vi "Instrument Manager Loop.vi"(8 "System Control":refnum<queue>, 11 "Instrument Manager":refnum<queue>) -> (0 "error out":errorcluster)   [LabVIEW 2020, in "Omega Platinum Series Plugin.lvlib" / "Instrument Manager.lvlib"]
uses:
  Instrument Manager/Instrument Manager.lvlib
  support/Message Queue/Message Cluster.ctl
  Instrument Manager/Instrument State.ctl
  <vilib>/Utility/error.llb/Error Cluster From Error Code.vi
  <vilib>/ErrorRing/Error Ring.xnode
  support/Message Queue/Message Queue.lvlib
  Omega Platinum Series Plugin.lvlib
  <instrlib>/RxnRover/OmegaPlatinumSeriesDriver/Omega Platinum Series.lvlib
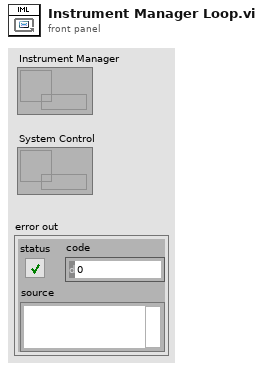
[diagram p1: front panel]
types:
  T1 = typedef "Omega Platinum Series Plugin.lvlib/Instrument Manager.lvlib/Instrument State.ctl" = cluster{"VISA Resource":refnum<visa-resource-name>, "Setpoint":dbl, "Running":bool, "Running Since":timestamp, "Data Point":cluster{"Time Stamp":timestamp, "Value":dbl}, "Sampling Rate (sec/sample)":dbl}
  T2 = typedef "Omega Platinum Series.lvlib/System State.ctl" = enum16{"LOAD", "IDLE", "INPUT_ADJUST", "CONTROL_ADJUST", "MODIFY", "WAIT", "RUN", "STANDBY", "STOP", "PAUSE", "FAULT", "SHUTDOWN", "AUTOTUNE"}
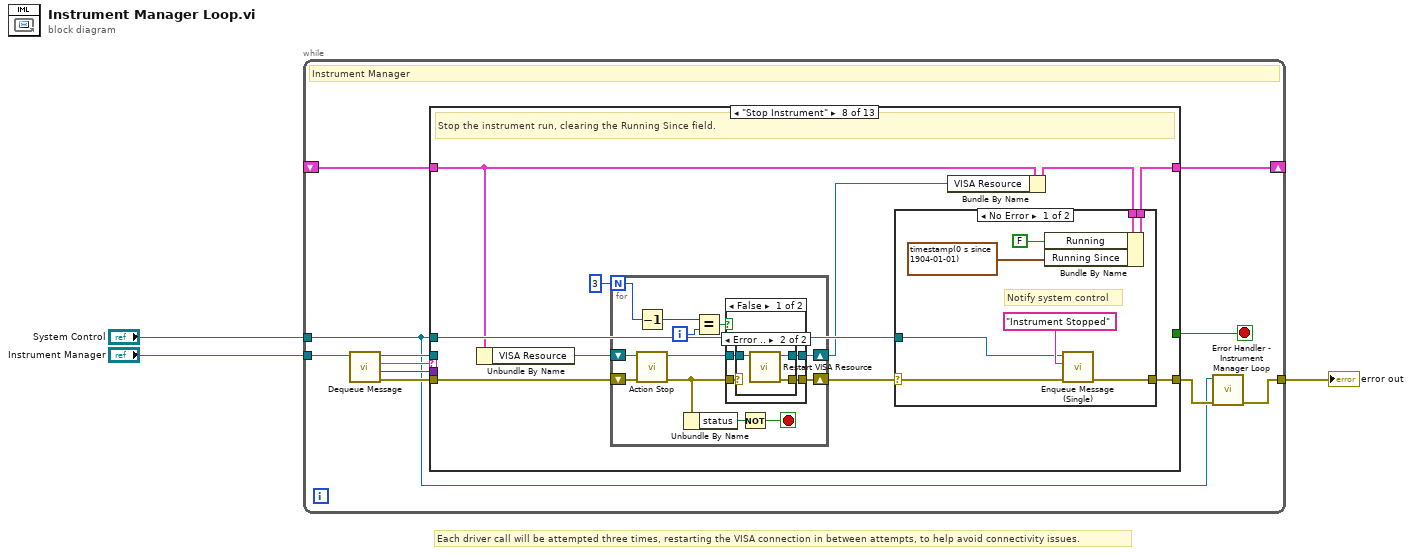
[diagram p0: block diagram]
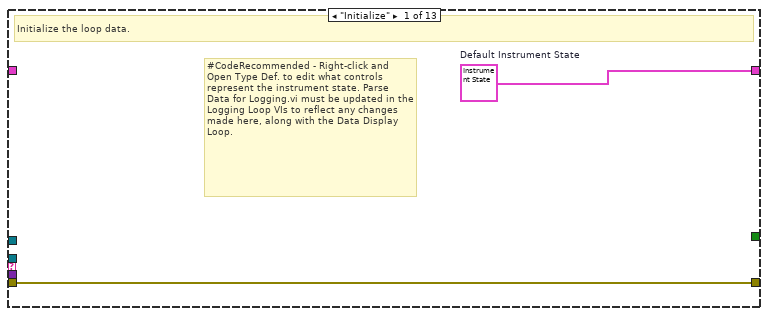
[diagram p2: hidden frame]
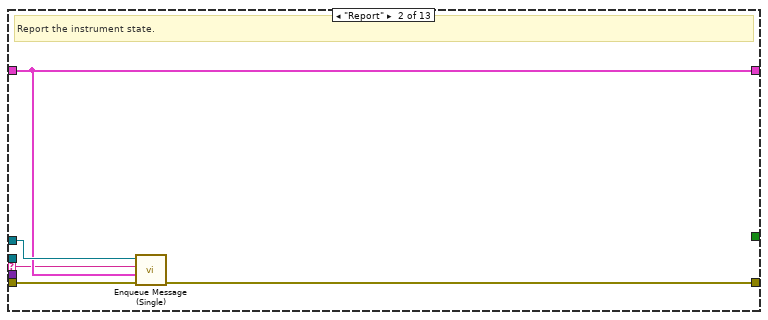
[diagram p3: hidden frame]
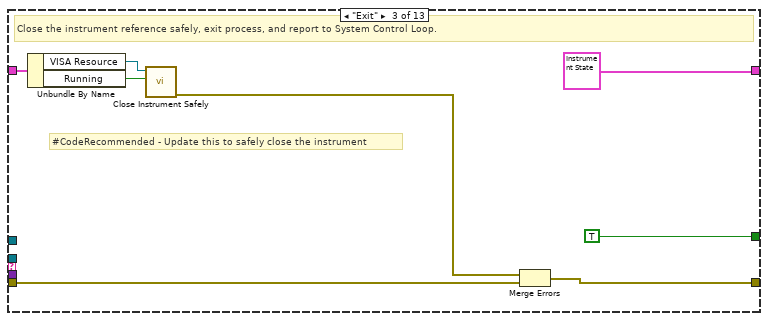
[diagram p4: hidden frame]
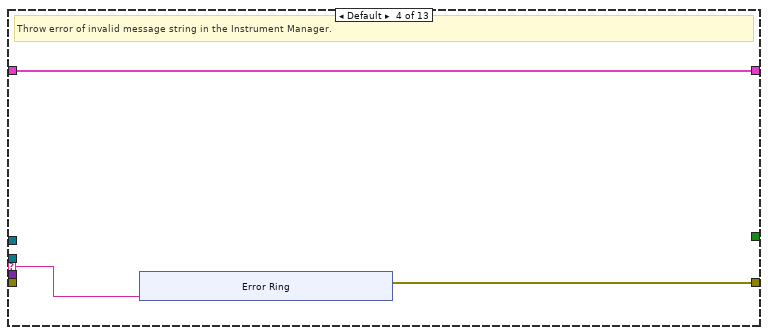
[diagram p5: hidden frame]
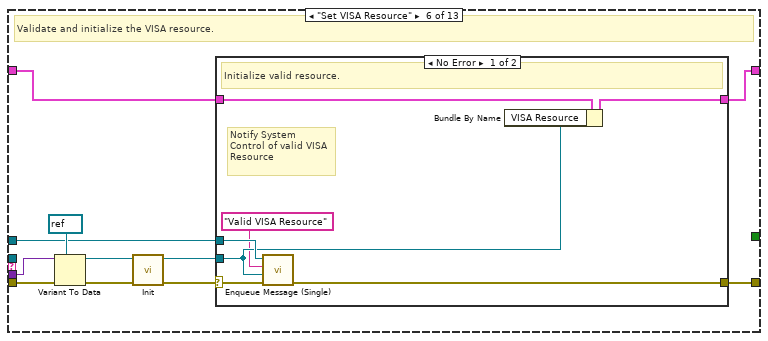
[diagram p7: hidden frame]
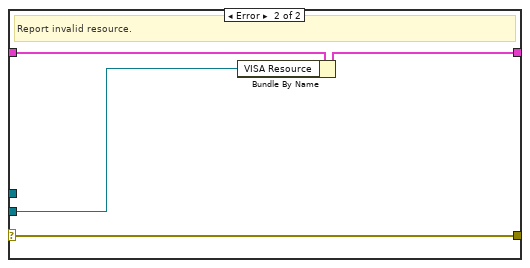
[diagram p8: hidden frame]
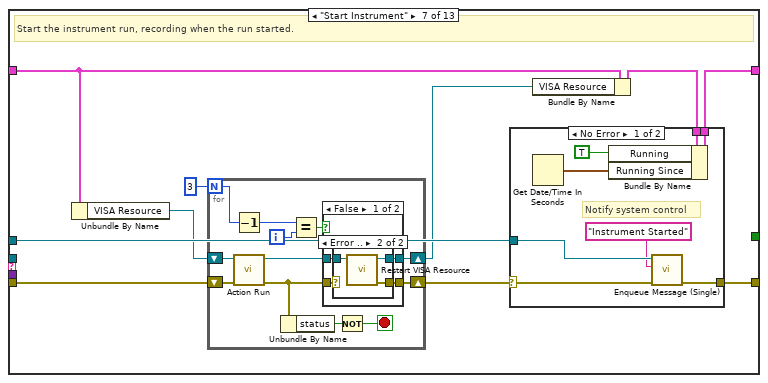
[diagram p9: hidden frame]
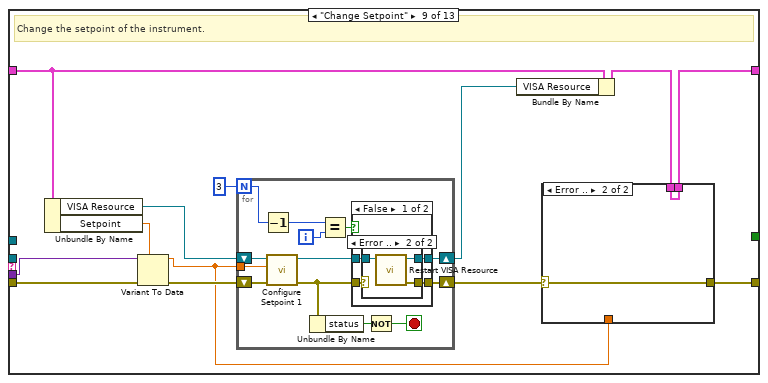
[diagram p16: hidden frame]
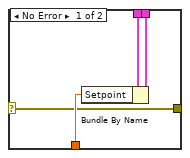
[diagram p17: hidden frame]
diagram:
  # "Each driver call will be attempted three times, restarting the VISA connection in between attempts, to help avoid connectivity issues."
  n1 = while {
    tunnel: "Instrument Manager" -> [w14]
    tunnel: "System Control" -> [w5]
    tunnel: [w8] -> w1
    shift-right: [w7] -> _
    shift-left: _ -> [w4]
    stop <- w6 stop-if-true
    # "Instrument Manager"
    n2 = call "Dequeue Message.vi"("Message Queue"=w14) -> ("error out"=w10:errorcluster, "Message Data"=w11:variant, "Message"=w13:string, "dup Message Queue"=w12:refnum<queue>)  [unwired: 7 in]
    n3 = case shown="\"Stop Instrument\"" w13 {
      selector: w13 -> [_ w17 _ w31 _ _ _ _ _ _ _ _ _]
      tunnel: w12 -> [_ _ _ _ _ _ _ _ _ _ _ _ _]
      tunnel: w5 -> [_ w20 _ _ _ w42 w72 w115 _ _ _ _ _]
      tunnel: w11 -> [_ _ _ _ _ w49 _ _ w161 _ _ _ _]
      tunnel: w10 -> [w15 w21 w24 _ w40 w48 w68 w112 w156 w194 w203 w239 w284]
      tunnel: [w15 w19 w23 w30 w40 w52 w73 w116 w152 w194 w202 w237 w280] -> w9
      tunnel: w4 -> [_ w18 w29 w32 w41 w51 w70 w113 w160 w193 w197 w236 w279]
      tunnel: [w16 w18 T1 {"VISA Resource"="", "Setpoint"=0.0, "Running"=FALSE, "Running Since"=timestamp(0 s since 1904-01-01), "Data Point"={"Time Stamp"=timestamp(0 s since 1904-01-01), "Value"=0.0}, "Sampling Rate (sec/sample)"=0.0} w32 w41 w50 w71 w114 w162 w193 w199 w243 w286] -> w7
      tunnel: [_ _ TRUE _ _ _ _ _ _ _ _ _ _] -> w6
      frame "Initialize" {
        w16 = T1 {"VISA Resource"="", "Setpoint"=0.0, "Running"=FALSE, "Running Since"=timestamp(0 s since 1904-01-01), "Data Point"={"Time Stamp"=timestamp(0 s since 1904-01-01), "Value"=0.0}, "Sampling Rate (sec/sample)"=0.0}  # Default Instrument State
        # "#CodeRecommended - Right-click and Open Type Def. to edit what controls represent the instrument state. Parse Data for Logging.vi must be updated in the Logging Loop VIs to reflect any changes made here, along with the Data Display Loop."
        # "Initialize the loop data."
      }
      frame "Report" {
        # "Report the instrument state."
        n4 = call "Enqueue Message (Single).vi"("error in (no error)"=w21, "Message Data"=w18, "Message"=w17, "Message Queue"=w20) -> ("error out"=w19:errorcluster)  [unwired: 6 in, 1 out]
      }
      frame "Exit" {
        # "#CodeRecommended - Update this to safely close the instrument"
        # "Close the instrument reference safely, exit process, and report to System Control Loop."
        n5 = Unbundle By Name(w29) -> ("VISA Resource"=w27:refnum<visa-resource-name>, "Running"=w28:bool)
        n6 = call "Close Instrument Safely.vi"("Running (F)"=w28, "VISA Refnum in"=w27) -> ("error out"=w22:errorcluster)  [unwired: 9 in]
        n7 = Merge Errors(w22, w24) -> (w23:errorcluster)
      }
      frame Default {
        # "Throw error of invalid message string in the Instrument Manager."
        n8 = xnode "Error Ring"("parameter 0"=w31) -> ("error out"=w30:errorcluster)
      }
      frame "--- Copy This Frame ---" {
        # "Copy this frame and add responses to instrument specific messages."
      }
      frame "Set VISA Resource" {
        # "Validate and initialize the VISA resource."
        n9 = Variant To Data(error in=w48, type=refnum<visa-resource-name> refnum, Variant=w49) -> (data=w46:refnum<visa-resource-name>, error out=w47:errorcluster)
        n10 = call "Init.vi"("error in (no error)"=w47, "VISA resource in"=w46) -> ("error out"=w43:errorcluster, "VISA resource out"=w44:refnum<visa-resource-name>)  [unwired: 8 in]
        n11 = case shown="No Error" w43 {
          selector: w43 -> [w58 w60]
          tunnel: w44 -> [w55 w61]
          tunnel: [w57 w60] -> w52
          tunnel: w51 -> [w59 w63]
          tunnel: [w53 w62] -> w50
          tunnel: w42 -> [w56 _]
          frame No Error {
            # "Notify System Control of valid VISA Resource"
            # "Initialize valid resource."
            n12 = call "Enqueue Message (Single).vi"("error in (no error)"=w58, "Message Data"=w55, "Message"="Valid VISA Resource", "Message Queue"=w56) -> ("error out"=w57:errorcluster)  [unwired: 6 in, 1 out]
            n13 = Bundle By Name(cluster=w59, "VISA Resource"=w55) -> (w53:T1)
          }
          frame Error {
            # "Report invalid resource."
            n14 = Bundle By Name(cluster=w63, "VISA Resource"=w61) -> (w62:T1)
          }
        }
      }
      frame "Start Instrument" {
        # "Start the instrument run, recording when the run started."
        n15 = Unbundle By Name(w70) -> ("VISA Resource"=w67:refnum<visa-resource-name>)
        n16 = for {
          N: 3 -> [w89]
          shift-right: [w92] -> w66
          shift-left: w68 -> [w86]
          shift-right: [w95] -> w64
          shift-left: w67 -> [w87]
          i -> [w90]
          stop <- w93 stop-if-true
          n17 = Decrement(x=w89) -> (x-1=w88:i32)
          n18 = call <instrlib>:"Action Run.vi"("error in (no error)"=w86, "VISA resource name (in)"=w87) -> ("error out"=w85:errorcluster, "VISA resource name (out)"=w84:refnum<visa-resource-name>)  [unwired: 7 in, 1 out]
          n19 = Unbundle By Name(w85) -> ("status"=w94:bool)
          n20 = Equal?(x=w88, y=w90) -> (x = y?=w91:bool)
          n21 = case shown="False" w91 {
            tunnel: w84 -> [w99 w106]
            tunnel: [w98 w106] -> w95
            tunnel: w85 -> [w97 w105]
            tunnel: [w96 w105] -> w92
            frame False {
              n22 = case shown="Error .." w97 {
                selector: w97 -> [w100 _]
                tunnel: w99 -> [w101 w104]
                tunnel: [w101 w103] -> w98
                tunnel: [w100 w102] -> w96
                frame No Error {
                }
                frame Error {
                  n23 = call "Restart VISA Resource.vi"("VISA Refnum in"=w104) -> ("error out"=w102:errorcluster, "VISA Refnum out"=w103:refnum<visa-resource-name>)  [unwired: 9 in]
                }
              }
            }
            frame True {
            }
          }
          n24 = Not(x=w94) -> (.not. x?=w93:bool)
        }
        n25 = Bundle By Name(cluster=w70, "VISA Resource"=w64) -> (w65:T1)
        n26 = case shown="No Error" w66 {
          selector: w66 -> [w74 w83]
          tunnel: [w81 w83] -> w73
          tunnel: w72 -> [w80 _]
          tunnel: [w78 w82] -> w71
          tunnel: w65 -> [w75 w82]
          frame No Error {
            # "Notify system control"
            n27 = Get Date/Time In Seconds() -> (seconds since 1Jan1904=w76:timestamp)
            n28 = Bundle By Name(cluster=w75, "Running"=TRUE, "Running Since"=w76) -> (w78:T1)
            n29 = call "Enqueue Message (Single).vi"("error in (no error)"=w74, "Message"="Instrument Started", "Message Queue"=w80) -> ("error out"=w81:errorcluster)  [unwired: 7 in, 1 out]
          }
          frame Error {
          }
        }
      }
      frame "Stop Instrument" {
        # "Stop the instrument run, clearing the Running Since field."
        n30 = Unbundle By Name(w113) -> ("VISA Resource"=w111:refnum<visa-resource-name>)
        n31 = for {
          N: 3 -> [w132]
          shift-right: [w135] -> w108
          shift-left: w112 -> [w130]
          shift-right: [w138] -> w109
          shift-left: w111 -> [w127]
          i -> [w133]
          stop <- w136 stop-if-true
          n32 = Decrement(x=w132) -> (x-1=w131:i32)
          n33 = call <instrlib>:"Action Stop.vi"("error in (no error)"=w130, "VISA resource name (in)"=w127) -> ("error out"=w129:errorcluster, "VISA resource name (out)"=w128:refnum<visa-resource-name>)  [unwired: 7 in, 1 out]
          n34 = Unbundle By Name(w129) -> ("status"=w137:bool)
          n35 = Equal?(x=w131, y=w133) -> (x = y?=w134:bool)
          n36 = case shown="False" w134 {
            tunnel: w128 -> [w142 w149]
            tunnel: [w141 w149] -> w138
            tunnel: w129 -> [w140 w148]
            tunnel: [w139 w148] -> w135
            frame False {
              n37 = case shown="Error .." w140 {
                selector: w140 -> [w143 _]
                tunnel: w142 -> [w144 w147]
                tunnel: [w144 w146] -> w141
                tunnel: [w143 w145] -> w139
                frame No Error {
                }
                frame Error {
                  n38 = call "Restart VISA Resource.vi"("VISA Refnum in"=w147) -> ("error out"=w145:errorcluster, "VISA Refnum out"=w146:refnum<visa-resource-name>)  [unwired: 9 in]
                }
              }
            }
            frame True {
            }
          }
          n39 = Not(x=w137) -> (.not. x?=w136:bool)
        }
        n40 = Bundle By Name(cluster=w113, "VISA Resource"=w109) -> (w110:T1)
        n41 = case shown="No Error" w108 {
          selector: w108 -> [w117 w125]
          tunnel: [w118 w125] -> w116
          tunnel: w115 -> [w123 _]
          tunnel: [w122 w126] -> w114
          tunnel: w110 -> [w119 w126]
          frame No Error {
            # "Notify system control"
            n42 = Bundle By Name(cluster=w119, "Running"=FALSE, "Running Since"=timestamp(0 s since 1904-01-01)) -> (w122:T1)
            n43 = call "Enqueue Message (Single).vi"("error in (no error)"=w117, "Message"="Instrument Stopped", "Message Queue"=w123) -> ("error out"=w118:errorcluster)  [unwired: 7 in, 1 out]
          }
          frame Error {
          }
        }
      }
      frame "Change Setpoint" {
        # "Change the setpoint of the instrument."
        n44 = Unbundle By Name(w160) -> ("VISA Resource"=w157:refnum<visa-resource-name>, "Setpoint"=w159:dbl)
        n45 = Variant To Data(error in=w156, type=w159, Variant=w161) -> (data=w153:dbl, error out=w155:errorcluster)
        n46 = for {
          N: 3 -> [w175]
          shift-right: [w178] -> w154
          shift-left: w155 -> [w171]
          shift-right: [w181] -> w150
          shift-left: w157 -> [w170]
          tunnel: w153 -> [w169]
          i -> [w176]
          stop <- w179 stop-if-true
          n47 = Decrement(x=w175) -> (x-1=w174:i32)
          n48 = call <instrlib>:"Configure Setpoint 1.vi"("error in (no error)"=w171, "Setpoint value"=w169, "VISA resource name (in)"=w170) -> ("error out"=w172:errorcluster, "VISA resource name (out)"=w173:refnum<visa-resource-name>)  [unwired: 6 in, 1 out]
          n49 = Unbundle By Name(w172) -> ("status"=w180:bool)
          n50 = Equal?(x=w174, y=w176) -> (x = y?=w177:bool)
          n51 = case shown="False" w177 {
            tunnel: w173 -> [w185 w192]
            tunnel: [w184 w192] -> w181
            tunnel: w172 -> [w183 w191]
            tunnel: [w182 w191] -> w178
            frame False {
              n52 = case shown="Error .." w183 {
                selector: w183 -> [w186 _]
                tunnel: w185 -> [w187 w190]
                tunnel: [w187 w189] -> w184
                tunnel: [w186 w188] -> w182
                frame No Error {
                }
                frame Error {
                  n53 = call "Restart VISA Resource.vi"("VISA Refnum in"=w190) -> ("error out"=w188:errorcluster, "VISA Refnum out"=w189:refnum<visa-resource-name>)  [unwired: 9 in]
                }
              }
            }
            frame True {
            }
          }
          n54 = Not(x=w180) -> (.not. x?=w179:bool)
        }
        n55 = Bundle By Name(cluster=w160, "VISA Resource"=w150) -> (w151:T1)
        n56 = case shown="Error .." w154 {
          selector: w154 -> [w163 w167]
          tunnel: [w166 w168] -> w162
          tunnel: w151 -> [w165 w168]
          tunnel: w153 -> [w164 _]
          tunnel: [w163 w167] -> w152
          frame No Error {
            n57 = Bundle By Name(cluster=w165, "Setpoint"=w164) -> (w166:T1)
          }
          frame Error {
          }
        }
      }
      frame "--- Copy for Get State Messages ---" {
        # "#CodeNeeded - Use the Bundle by Name function to bundle the new state value into the Instrument State cluster."
        # "#CodeNeeded - Add instrument driver call to query the instrument state requested"
        # "Duplicate this case for messages cases that will query the instrument state."
      }
      frame "Run State" {
        # "Query the run state of the instrument."
        n58 = Unbundle By Name(w197) -> ("VISA Resource"=w201:refnum<visa-resource-name>)
        n59 = for {
          N: 3 -> [w205]
          tunnel: [w214] -> w200
          shift-right: [w208] -> w202
          shift-left: w203 -> [w216]
          shift-right: [w212] -> w195
          shift-left: w201 -> [w215]
          i -> [w206]
          stop <- w210 stop-if-true
          n60 = Decrement(x=w205) -> (x-1=w204:i32)
          n61 = call <instrlib>:"Status System State.vi"("error in (no error)"=w216, "VISA resource name (in)"=w215) -> ("error out"=w209:errorcluster, "System State"=w214:T2, "VISA resource name (out)"=w213:refnum<visa-resource-name>)  [unwired: 7 in]
          n62 = Unbundle By Name(w209) -> ("status"=w211:bool)
          n63 = Equal?(x=w204, y=w206) -> (x = y?=w207:bool)
          n64 = case shown="False" w207 {
            tunnel: w213 -> [w220 w227]
            tunnel: [w219 w227] -> w212
            tunnel: w209 -> [w218 w226]
            tunnel: [w217 w226] -> w208
            frame False {
              n65 = case shown="Error .." w218 {
                selector: w218 -> [w221 _]
                tunnel: w220 -> [w222 w225]
                tunnel: [w222 w224] -> w219
                tunnel: [w221 w223] -> w217
                frame No Error {
                }
                frame Error {
                  n66 = call "Restart VISA Resource.vi"("VISA Refnum in"=w225) -> ("error out"=w223:errorcluster, "VISA Refnum out"=w224:refnum<visa-resource-name>)  [unwired: 9 in]
                }
              }
            }
            frame True {
            }
          }
          n67 = Not(x=w211) -> (.not. x?=w210:bool)
        }
        n68 = Bundle By Name(cluster=w197, "VISA Resource"=w195) -> (w196:T1)
        n69 = case shown="\"RUN\", \"AUTOTUNE\"" w200 {
          tunnel: w196 -> [w229 w233]
          tunnel: [w230 w232] -> w199
          frame "IDLE", Default {
            n70 = Bundle By Name(cluster=w229, "Running"=FALSE) -> (w230:T1)
          }
          frame "RUN", "AUTOTUNE" {
            n71 = Bundle By Name(cluster=w233, "Running"=TRUE) -> (w232:T1)
          }
        }
      }
      frame "Temperature" {
        # "Query the temperature reading of the instrument."
        n72 = Unbundle By Name(w236) -> ("VISA Resource"=w241:refnum<visa-resource-name>)
        n73 = for {
          N: 3 -> [w259]
          shift-right: [w262] -> w238
          shift-left: w239 -> [w256]
          shift-right: [w265] -> w234
          shift-left: w241 -> [w257]
          tunnel: [w253] -> w240
          i -> [w260]
          stop <- w263 stop-if-true
          n74 = Decrement(x=w259) -> (x-1=w258:i32)
          n75 = call <instrlib>:"Status Read Temperature.vi"("error in (no error)"=w256, "VISA resource name (in)"=w257) -> ("error out"=w255:errorcluster, "Temperature"=w253:string, "VISA resource name (out)"=w254:refnum<visa-resource-name>)  [unwired: 7 in]
          n76 = Unbundle By Name(w255) -> ("status"=w264:bool)
          n77 = Equal?(x=w258, y=w260) -> (x = y?=w261:bool)
          n78 = case shown="False" w261 {
            tunnel: w254 -> [w269 w276]
            tunnel: [w268 w276] -> w265
            tunnel: w255 -> [w267 w275]
            tunnel: [w266 w275] -> w262
            frame False {
              n79 = case shown="Error .." w267 {
                selector: w267 -> [w270 _]
                tunnel: w269 -> [w271 w274]
                tunnel: [w271 w273] -> w268
                tunnel: [w270 w272] -> w266
                frame No Error {
                }
                frame Error {
                  n80 = call "Restart VISA Resource.vi"("VISA Refnum in"=w274) -> ("error out"=w272:errorcluster, "VISA Refnum out"=w273:refnum<visa-resource-name>)  [unwired: 9 in]
                }
              }
            }
            frame True {
            }
          }
          n81 = Not(x=w264) -> (.not. x?=w263:bool)
        }
        n82 = Bundle By Name(cluster=w236, "VISA Resource"=w234) -> (w235:T1)
        n83 = case shown="No Error" w238 {
          selector: w238 -> [w244 w252]
          tunnel: [w250 w251] -> w243
          tunnel: w235 -> [w247 w251]
          tunnel: w240 -> [w245 _]
          tunnel: [w244 w252] -> w237
          frame No Error {
            n84 = Fract/Exp String To Number(string=w245) -> (number=w246:dbl)  [unwired: 3 in, 1 out]
            n85 = Get Date/Time In Seconds() -> (seconds since 1Jan1904=w249:timestamp)
            n86 = Bundle("seconds since 1Jan1904"=w249, w246) -> (w248:cluster{"seconds since 1Jan1904":timestamp, dbl})  [unwired: 1 in]
            n87 = Bundle By Name(cluster=w247, "Data Point"=w248) -> (w250:T1)
          }
          frame Error {
          }
        }
      }
      frame "Setpoint" {
        # "Query the setpoint of the instrument."
        n88 = Unbundle By Name(w279) -> ("VISA Resource"=w283:refnum<visa-resource-name>)
        n89 = for {
          N: 3 -> [w300]
          tunnel: [w294] -> w282
          shift-right: [w303] -> w281
          shift-left: w284 -> [w297]
          shift-right: [w306] -> w277
          shift-left: w283 -> [w298]
          i -> [w301]
          stop <- w304 stop-if-true
          n90 = call <instrlib>:"Status Setpoint 1.vi"("error in (no error)"=w297, "VISA resource name (in)"=w298) -> ("error out"=w296:errorcluster, "Setpoint 1"=w294:string, "VISA resource name (out)"=w295:refnum<visa-resource-name>)  [unwired: 7 in]
          n91 = Decrement(x=w300) -> (x-1=w299:i32)
          n92 = Unbundle By Name(w296) -> ("status"=w305:bool)
          n93 = Equal?(x=w299, y=w301) -> (x = y?=w302:bool)
          n94 = case shown="False" w302 {
            tunnel: w295 -> [w310 w317]
            tunnel: [w309 w317] -> w306
            tunnel: w296 -> [w308 w316]
            tunnel: [w307 w316] -> w303
            frame False {
              n95 = case shown="Error .." w308 {
                selector: w308 -> [w311 _]
                tunnel: w310 -> [w312 w315]
                tunnel: [w312 w314] -> w309
                tunnel: [w311 w313] -> w307
                frame No Error {
                }
                frame Error {
                  n96 = call "Restart VISA Resource.vi"("VISA Refnum in"=w315) -> ("error out"=w313:errorcluster, "VISA Refnum out"=w314:refnum<visa-resource-name>)  [unwired: 9 in]
                }
              }
            }
            frame True {
            }
          }
          n97 = Not(x=w305) -> (.not. x?=w304:bool)
        }
        n98 = Bundle By Name(cluster=w279, "VISA Resource"=w277) -> (w278:T1)
        n99 = case shown="No Error" w281 {
          selector: w281 -> [w287 w292]
          tunnel: w278 -> [w291 w293]
          tunnel: [w290 w293] -> w286
          tunnel: w282 -> [w288 _]
          tunnel: [w287 w292] -> w280
          frame No Error {
            n100 = Fract/Exp String To Number(string=w288) -> (number=w289:dbl)  [unwired: 3 in, 1 out]
            n101 = Bundle By Name(cluster=w291, "Setpoint"=w289) -> (w290:T1)
          }
          frame Error {
          }
        }
      }
    }
    n102 = call "Error Handler - Instrument Manager Loop.vi"("error in (no error)"=w9, "Message Queue"=w5) -> ("dup error in"=w8:errorcluster)  [unwired: 8 in, 1 out]
  }
  "error out" <- w1
